vi "Actor Core.vi"(8 "error in":errorcluster, 11 "TabbedViewManager In":refnum<class "TabbedViewManager.lvclass">) -> (0 "error out":errorcluster, 3 "Actor out":refnum<class "Actor.lvclass">)   [LabVIEW 2020, in "MVA Framework.lvlib" / "TabbedViewManager.lvlib" / "TabbedViewManager.lvclass"]
doc: "(<B>Filename</B>: Actor Framework.lvlib:Actor.lvclass:Actor Core.vi)\n\nReceives messages to the actor, reacts to them, and initiates any error handling that may shut the actor down.\n\nDescendant classes may override this VI to append parallel tasks for the actor to complete while it handles messages. Overrides use the Call Parent Method node.\n\n<License>\nCopyright © 2017 Composed Systems, LLC | All rights reserved\nwww.composed.io\n\nAuthor: Ethan Stern <ethan.stern@composed.io>\n\nThis software is provided \"AS IS\" WITHOUT WARRANTIES, either express or implied, AND IS FOR EDUCATIONAL PURPOSES ONLY.\n</License>"
uses:
  TabbedViewManager.lvclass
  TabbedViewManager.lvclass/TabbedViewManager.ctl
  <vilib>/ActorFramework/Actor/Actor.lvclass
  TabbedViewManager Messages/Set View by Tab Index Msg/Set View by Tab Index Msg.lvclass
  modules/mva-viewable/Source/IViewable/ProtectedSubpanel/ProtectedSubpanel.lvclass
  modules/mva-viewable/Source/IViewManager/IViewManager/IViewManager.lvclass
  C:/Program Files/National Instruments/LabVIEW 2020/vi.lib/ActorFramework/Actor/Actor.lvclass
panel:
  in  "Tab Control":T1(tab)
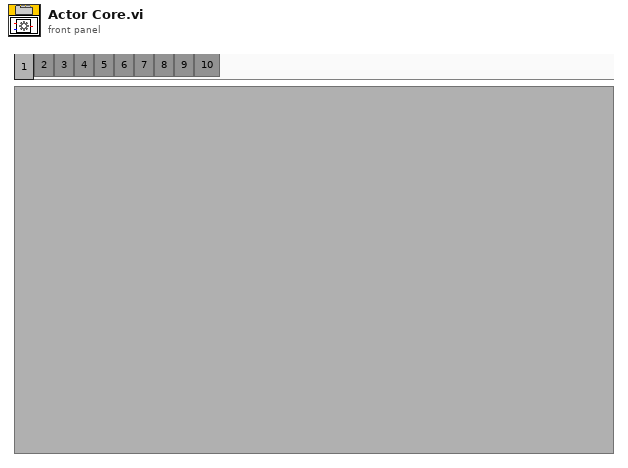
[diagram p1: front panel]
types:
  T1 = enum32{"1", "2", "3", "4", "5", "6", "7", "8", "9", "10"}
  T2 = typedef "MVA Framework.lvlib/IViewable.lvlib/ProtectedSubpanel.lvclass/Protected Subpanel Reference.ctl" = refnum<data-value>
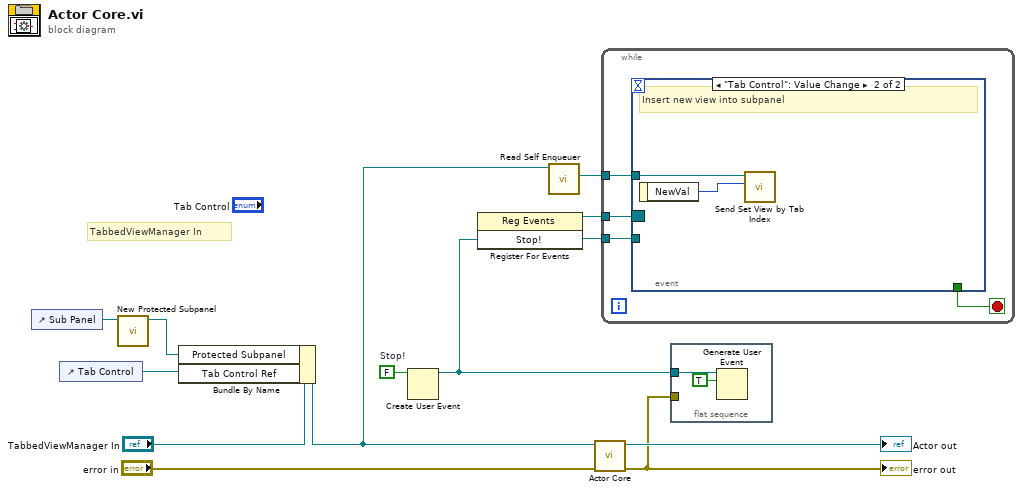
[diagram p0: block diagram]
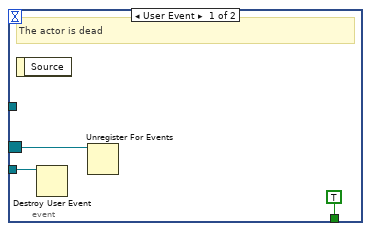
[diagram p2: hidden frame]
diagram:
  w2 = FALSE  # Stop!
  # "TabbedViewManager In"
  n1 = control-ref of="Sub Panel"() -> (w1:refnum<vi>)
  n2 = control-ref of="Tab Control"() -> (w10:refnum<vi>)
  n3 = call "New Protected Subpanel.vi"("SubPnl Refnum"=w1) -> ("Protected Subpanel"=w4:T2)  [unwired: 9 in, 1 out]
  n4 = Bundle By Name(cluster="TabbedViewManager In", "Protected Subpanel"=w4, "Tab Control Ref"=w10) -> (w7:refnum<class "TabbedViewManager.lvclass">)
  n5 = Create User Event(user event datatype=w2) -> (user event=w8:refnum<user-event>)  [unwired: 1 in, 1 out]
  n6 = register-events(w8) -> (reference out=w9:refnum<event-registration>)  [unwired: 2 in, 1 out]
  n7 = call <vilib>:"Read Self Enqueuer.vi"("Actor"=w7) -> ("Self Enqueuer"=w6:refnum<class "Message Enqueuer.lvclass">)  [unwired: 10 in]
  n8 = call-parent "Actor Core.vi"("error in"="error in", "IViewable In"=w7) -> ("error out"=w5:errorcluster, "Actor out"=→"Actor out":refnum<class "Actor.lvclass">)  [unwired: 8 in]
  "error out" <- w5
  n9 = while {
    tunnel: w9 -> [w16]
    tunnel: w8 -> [w15]
    tunnel: w6 -> [w13]
    stop <- w14 stop-if-true
    n10 = event shown="[1] \"Tab Control\": Value Change" {
      selector: w16 -> [w18 _]
      dyn-events: _ -> [_ _]
      timeout: _ -> [_ _]
      tunnel: w15 -> [w19 _]
      tunnel: [TRUE _] -> w14
      tunnel: w13 -> [_ w21]
      event User Event {
        # "The actor is dead"
        n11 = event-data() -> ()  [unwired: 1 in, 1 out]
        n12 = Destroy User Event(user event=w19) -> ()  [unwired: 1 in, 1 out]
        n13 = Unregister For Events(event registration refnum=w18) -> ()  [unwired: 1 in, 1 out]
      }
      event "Tab Control": Value Change {
        # "Insert new view into subpanel"
        n14 = event-data() -> ("NewVal"=w20:T1)  [unwired: 1 in]
        n15 = call "Send Set View by Tab Index.vi"("Index"=w20, "Message Enqueuer"=w21) -> ()  [unwired: 8 in, 2 out]
      }
    }
  }
  n16 = flat-sequence {
    tunnel: w8 -> [w23]
    tunnel: w5 -> [_]
    frame #0 {
      n17 = Generate User Event(user event=w23, event data cluster=TRUE ("event data")) -> ()  [unwired: 2 in, 2 out]
    }
  }
